vi "Sort ROI data.vi"(10 "Data for ticked ROI":T1=[{"Plot.Plot Name"="1: Point", "Data"={"X-Axis values"=array[43860 elements], "Y-Axis values (s)"=array[43860 elements]}, "Timeline data"={"X-Axis values"=[], "Y-Axis values (s)"=[]}, "Type"=enum."Mini-scan", "Points per cycle"=1, "ROI number"=0}], 11 "Data for ticked Groups":T1) -> (1 "POI  and POI groups raw data":T1, 2 "Miniscans and Mscn groups raw data":T1)   [LabVIEW 2020]
uses:
  xcontrol/Interface VIs/Interface typedefs/Interface-Data array.ctl
  xcontrol/Interface VIs/Interface typedefs/Interface-Data format definition.ctl
  xcontrol/Typedefs/Xctl-XY data type definition.ctl
  xcontrol/Typedefs/Xctrl-ROI type enum.ctl
  xcontrol/XGrapher.xctl
panel:
  # "<--- This can be used to reorder a concatenated array of any type containing miniscans first, followed by POI."
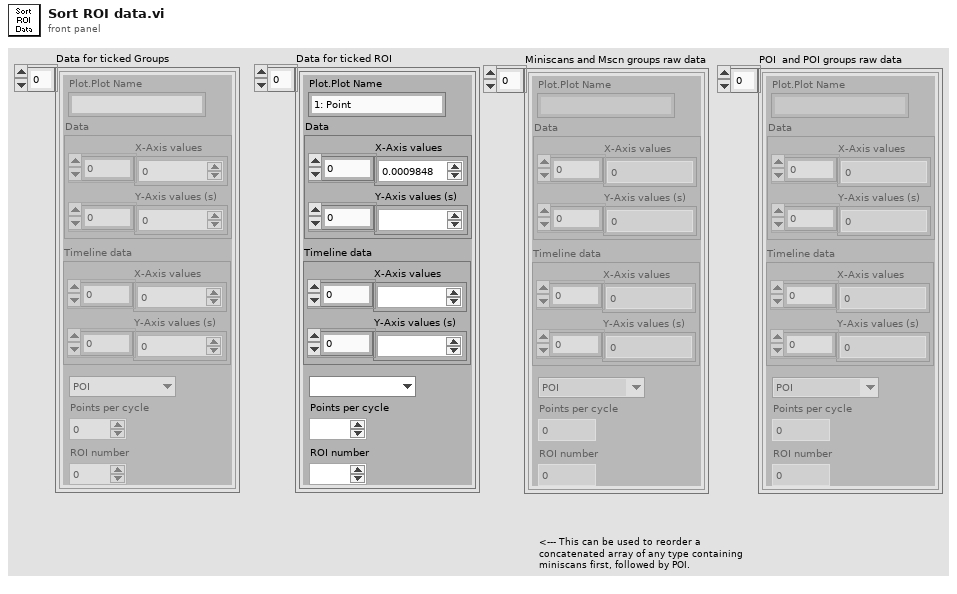
[diagram p1: front panel]
types:
  T1 = typedef "Interface-Data array.ctl" = T2[]
  T2 = typedef "Interface-Data format definition.ctl" = cluster{"Plot.Plot Name":string, "Data":T3, "Timeline data":T3, "Type":T4, "Points per cycle":u16, "ROI number":u16}
  T3 = typedef "XGrapher.xctl/Xctl-XY data type definition.ctl" = cluster{"X-Axis values":sgl[], "Y-Axis values (s)":sgl[]}
  T4 = typedef "Xctrl-ROI type enum.ctl" = enum16{"POI", "Mini-scan", "Group"}
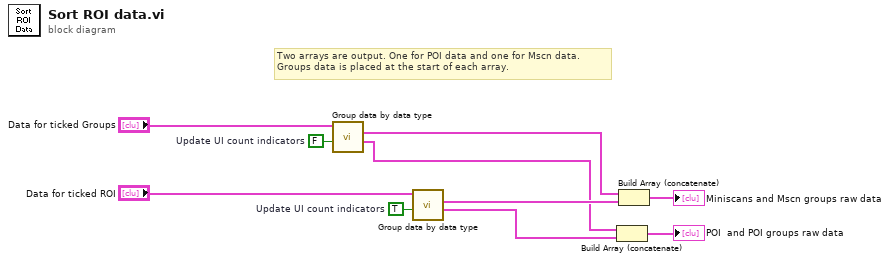
[diagram p0: block diagram]
diagram:
  w5 = FALSE  # Update UI count indicators
  w6 = TRUE  # Update UI count indicators
  # "Two arrays are output. One for POI data and one for Mscn data.\nGroups data is placed at the start of each array."
  n1 = call "Group data by data type.vi"("Update UI count indicators"=w5, "Raw data"="Data for ticked Groups") -> ("POI data"=w2:T1, "Miniscan data"=w4:T1)  [unwired: 7 in, 1 out]
  n2 = call "Group data by data type.vi"("Update UI count indicators"=w6, "Raw data"="Data for ticked ROI") -> ("POI data"=w1:T1, "Miniscan data"=w3:T1)  [unwired: 7 in, 1 out]
  n3 = Build Array (concatenate)(w2, w1) -> (→"POI  and POI groups raw data":T1)
  n4 = Build Array (concatenate)(w4, w3) -> (→"Miniscans and Mscn groups raw data":T1)
